vi "Get Value by Array (Boolean Value).vi"(8 "error in (no error)":errorcluster, 10 "Keys":string[](array[string]), 11 "JSON Object in":refnum<class "JSON Value.lvclass">) -> (0 "error out":errorcluster, 2 "value":bool)   [LabVIEW 2016, in "JSON Value.lvclass"]
uses:
  JSON Helper/JSON Value.lvclass
  Get Value by Array (JSON).vi
  JSON Boolean/Read value (Boolean).vi
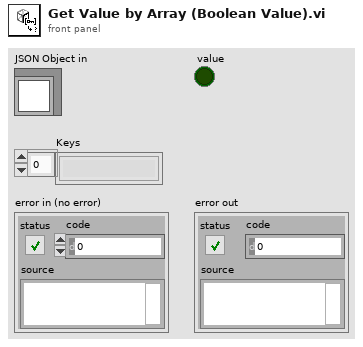
[diagram p1: front panel]
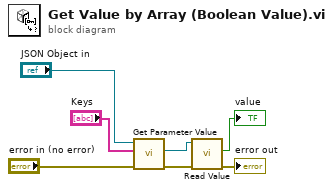
[diagram p0: block diagram]
diagram:
  n1 = call-poly "Get Parameter Value.vi"("error in (no error)"="error in (no error)", "Keys"="Keys", "JSON in"="JSON Object in") -> ("error out"=w5:errorcluster, "JSON out"=w4:refnum<class "JSON Value.lvclass">)  [unwired: 7 in]
  n2 = call-poly "Read Value.vi"("error in (no error)"=w5, "JSON Boolean in"=w4) -> ("error out"=→"error out":errorcluster, "value"=→"value":bool)  [unwired: 8 in]
